vi "集成干预数据插入.vi"(8 "error in (no error)":errorcluster, 11 "集成干预测试数据":T1={"时间"=timestamp(0 s since 1904-01-01), "参数"="", "数据类型"="N", "集成干预测试浓度值"=0.0, "集成干预前测试时间"=timestamp(0 s since 1904-01-01), "集成干预前测试浓度值"=0.0}) -> (0 "error out":errorcluster)   [LabVIEW 2016, in "质控单元V4.lvlib"]
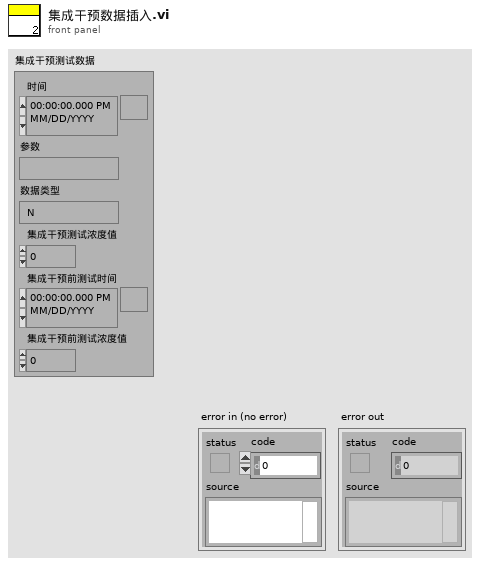
[diagram p1: front panel]
types:
  T1 = typedef "集成干预字段定义.ctl" = cluster{"时间":timestamp, "参数":string, "数据类型":string, "集成干预测试浓度值":dbl, "集成干预前测试时间":timestamp, "集成干预前测试浓度值":dbl}
  T2 = typedef "数据库类型.ctl" = enum16{"Access", "SQLite"}
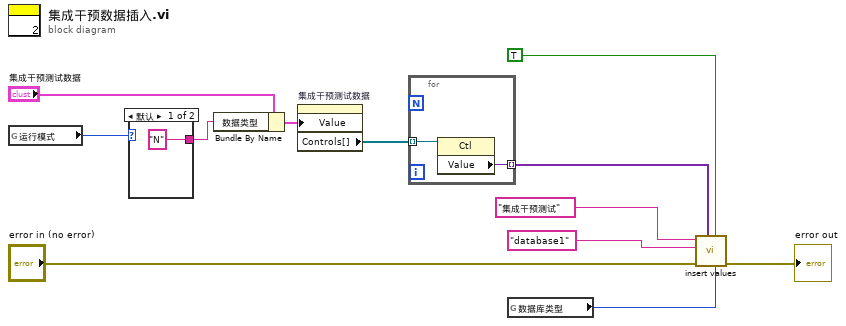
[diagram p0: block diagram]
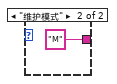
[diagram p2: hidden frame]
diagram:
  n1 = global read "系统交互.vi" "运行模式"() -> (w12:enum16{"维护模式", "常规模式", "应急模式", "质控模式"})
  n2 = case shown="默认" w12 {
    tunnel: ["N" "M"] -> w11
    frame Default {
    }
    frame "维护模式" {
    }
  }
  n3 = Bundle By Name(cluster="集成干预测试数据", "数据类型"=w11) -> (w2:T1)
  n4 = property on="集成干预测试数据" class="Clust (严格)"("Value"=w2) -> ("Controls[]"=w1:refnum<vi>[])  [unwired: 2 in, 2 out]
  n5 = for {
    tunnel: w1 -> [w16] mode=indexing
    tunnel: [w15] -> w5 mode=indexing
    n6 = property class="Ctl"(reference=w16) -> ("Value"=w15:variant)  [unwired: 1 in, 2 out]
  }
  n7 = global read "ZK断电保存全局变量.vi" "数据库类型"() -> (w8:T2)
  n8 = call "insert values.vi"("数据库类型"=w8, "是否创建唯一键"=TRUE, "data"=w5, "错误输入（无错误）"="error in (no error)", "database"="database1", "Tabe Name"="集成干预测试" ("table")) -> ("错误输出"=→"error out":errorcluster)  [unwired: 5 in]
